vi "AMC Multiple Targets Example 1.vi"() -> ()   [LabVIEW 2017]
uses:
  Tools/Keyed Array/Tools_KeyedArray KeyedArray.ctl
panel:
  in  "Servers":i32(listbox)
  in  "Get All Queues":bool
  in  "Target IP Address":string="10.0.18.197"
  in  "Queue":string
  in  "Verify Queue":bool
  in  "PingAll":bool
  out "Response":string
  in  "Ping":bool
  in  "Exit":bool
  out "Process":bool
  in  "Process":bool
  out "Status":string
  in  "Process":bool
  in  "Exit":bool
  in  "State Variables":T1
  # "Target1"
  # "Local Messages >>"
  # "Remote Messages >>"
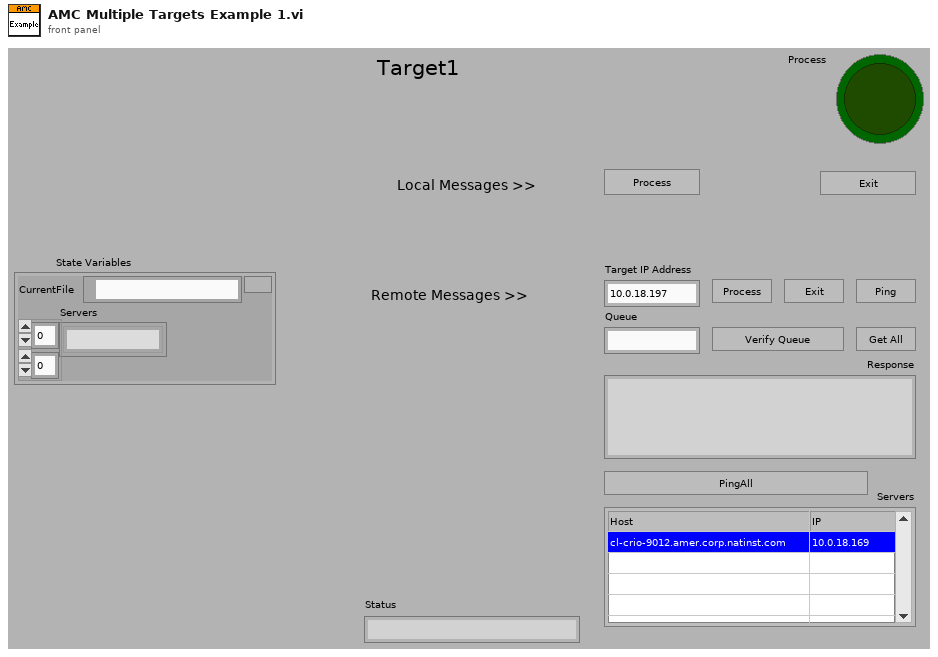
[diagram p1: front panel]
types:
  T1 = cluster{"CurrentFile":path, "Servers":string[][]}
  T2 = typedef "amc_Message Queue.ctl" = refnum<queue>
  T3 = typedef "Tools_KeyedArray KeyedArray.ctl" = cluster{"keys":string[], "values":string[]}
  T4 = typedef "LVPoint32TypeDef.ctl" = cluster{"Horizontal":i32, "Vertical":i32}
  T5 = typedef "LVRowAndColumnTypeDef.ctl" = cluster{"Row":i32, "Column":i32}
  T6 = typedef "amc_Message.ctl" = cluster{"Name":string, "Value":string, "Attributes":T3, "Receiver Host":string, "Receiver Process":string, "Source Host":string, "Source Process":string, "Priority Message":bool, "Acknowledge Message":bool}
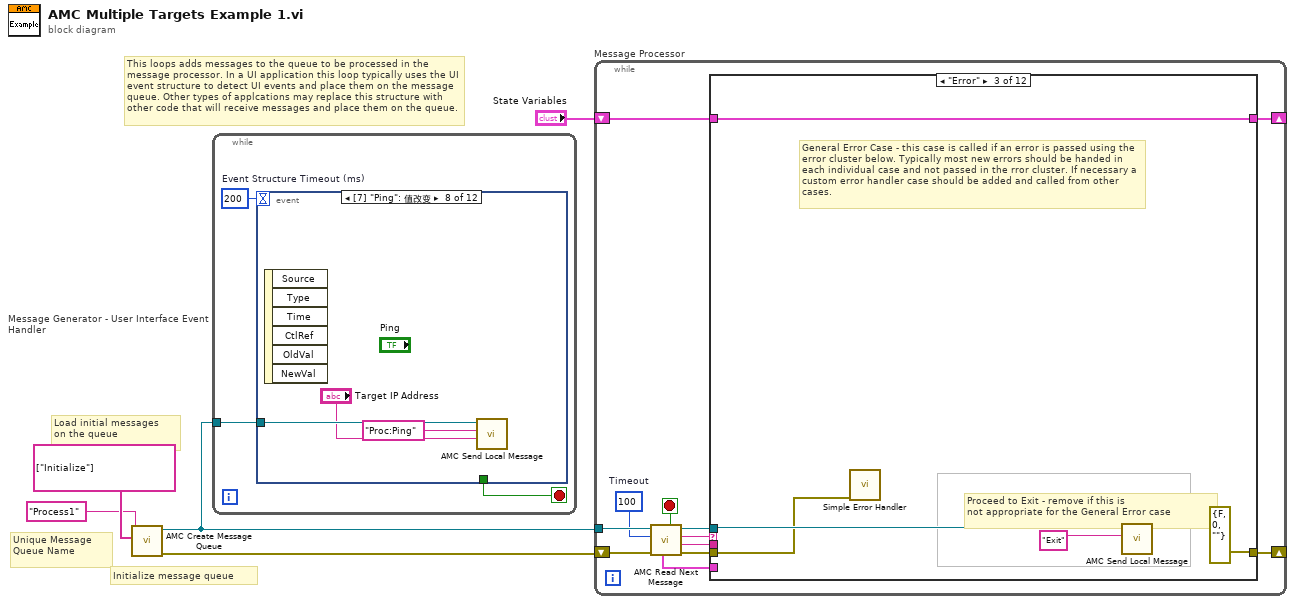
[diagram p0: block diagram]
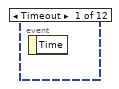
[diagram p2: hidden frame]
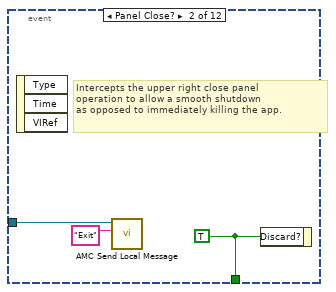
[diagram p3: hidden frame]
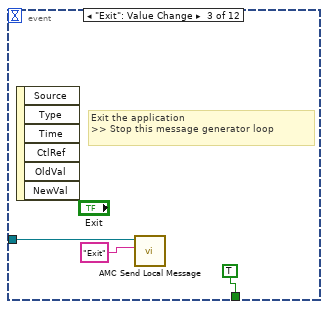
[diagram p4: hidden frame]
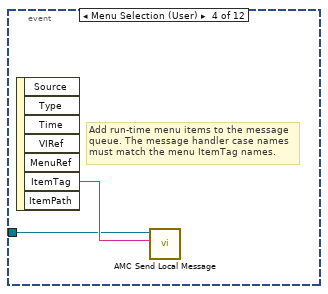
[diagram p5: hidden frame]
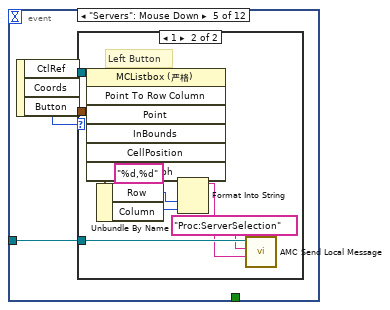
[diagram p6: hidden frame]
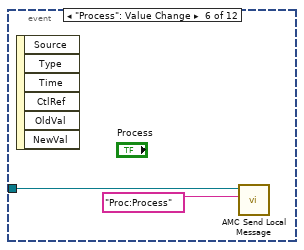
[diagram p8: hidden frame]
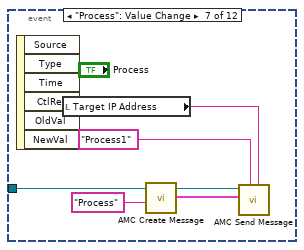
[diagram p9: hidden frame]
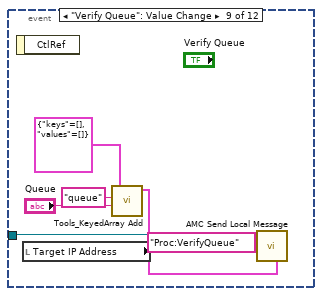
[diagram p10: hidden frame]
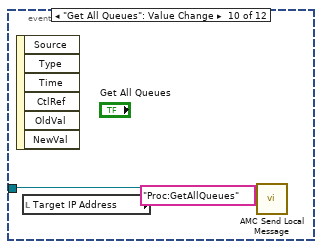
[diagram p11: hidden frame]
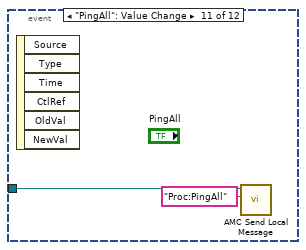
[diagram p12: hidden frame]
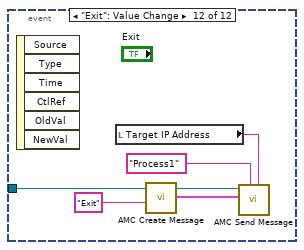
[diagram p13: hidden frame]
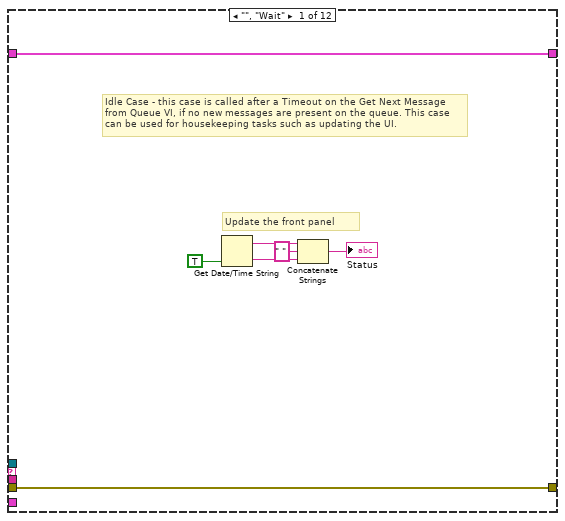
[diagram p14: hidden frame]
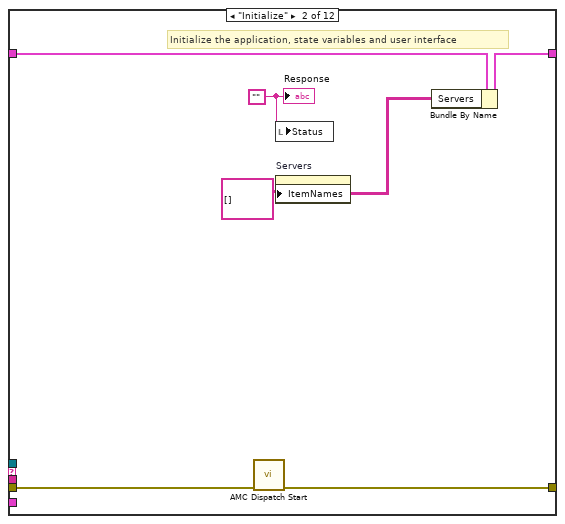
[diagram p15: hidden frame]
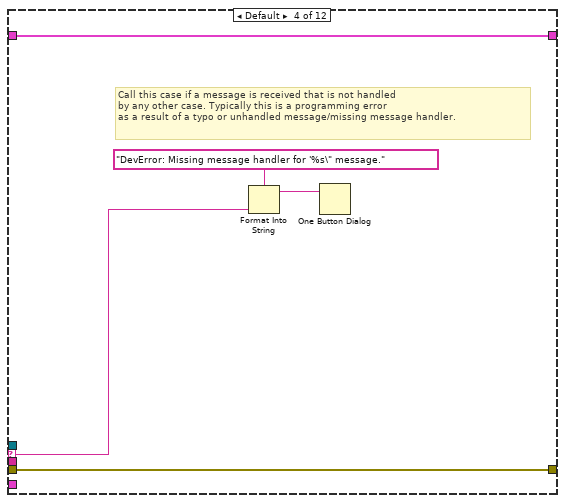
[diagram p16: hidden frame]
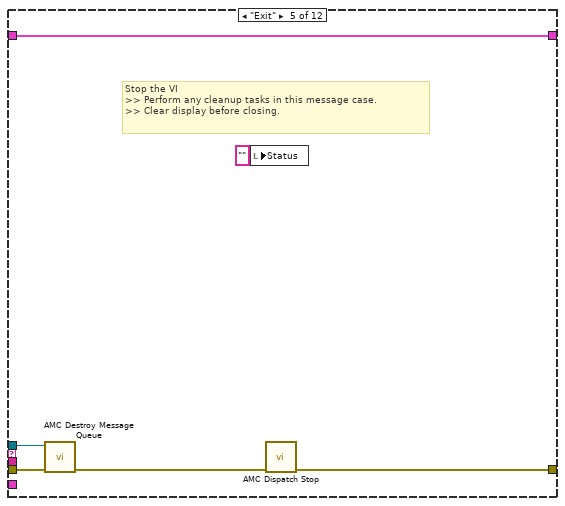
[diagram p17: hidden frame]
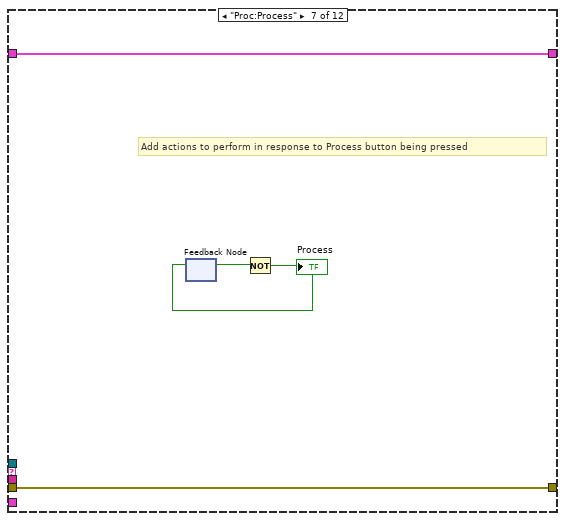
[diagram p19: hidden frame]
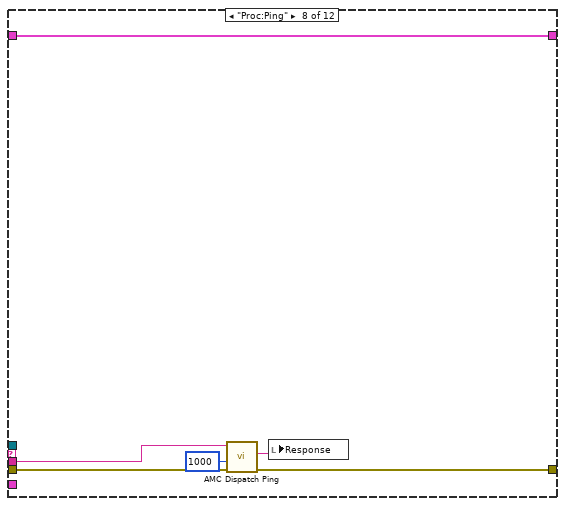
[diagram p20: hidden frame]
diagram:
  # "This loops adds messages to the queue to be processed in the message processor. In a UI application this loop typically uses the UI event structure to detect UI events and place them on the message queue. Other types of applcations may replace this structure with other code that will receive messages and place them on the queue."
  # "Initialize message queue"
  # "Unique Message\nQueue Name"
  # "Load initial messages\non the queue"
  n1 = call "AMC Create Message Queue.vi"("Initial Message Names"=string[] ["Initialize"], "Message Queue Name"="Process1" ("Message queue name (unnamed)")) -> ("error out"=w3:errorcluster, "Message Queue out"=w5:T2)  [unwired: 3 in, 5 out]
  n2 = while "Message Generator - User Interface Event Handler" {
    tunnel: w5 -> [w6]
    stop <- w7 stop-if-true
    w8 = 200  # Event Structure Timeout (ms)
    n3 = event shown="[7] \"Ping\": 值改变" {
      selector: _ -> [_ _ _ _ _ _ _ _ _ _ _ _]
      dyn-events: _ -> [_ _ _ _ _ _ _ _ _ _ _ _]
      timeout: w8 -> [_ _ _ _ _ _ _ _ _ _ _ _]
      tunnel: [_ w11 TRUE ("Discard?") _ _ _ _ _ _ _ _ _] -> w7
      tunnel: w6 -> [_ w9 w13 w15 w20 w31 w36 w39 w46 w49 w51 w56]
      event Timeout {
        n4 = event-data() -> ()  [unwired: 2 out]
      }
      event Panel Close? {
        w11 = TRUE ("Discard?")
        # "Intercepts the upper right close panel\noperation to allow a smooth shutdown\nas opposed to immediately killing the app."
        n5 = event-data() -> ()  [unwired: 4 out]
        n6 = call "AMC Send Local Message.vi"("Message Name"="Exit", "Message Queue in"=w9) -> ()  [unwired: 4 in, 6 out]
        n7 = event-data("Discard?"=w11) -> ()  [unwired: 1 in, 1 out]
      }
      event "Exit": Value Change {
        # "Exit the application\n>> Stop this message generator loop"
        n8 = event-data() -> ()  [unwired: 7 out]
        n9 = call "AMC Send Local Message.vi"("Message Name"="Exit", "Message Queue in"=w13) -> ()  [unwired: 4 in, 6 out]
      }
      event Menu Selection (User) {
        # "Add run-time menu items to the message\nqueue. The message handler case names must match the menu ItemTag names."
        n10 = event-data() -> ("ItemTag"=w16:string)  [unwired: 7 out]
        n11 = call "AMC Send Local Message.vi"("Message Name"=w16, "Message Queue in"=w15) -> ()  [unwired: 4 in, 6 out]
      }
      event "Servers": Mouse Down {
        n12 = event-data() -> ("CtlRef"=w19:refnum<vi>, "Coords"=w18:T4, "Button"=w17:u16)  [unwired: 1 out]
        n13 = case shown="1" w17 {
          tunnel: w20 -> [_ w29]
          tunnel: w19 -> [_ w27]
          tunnel: w18 -> [_ w26]
          frame Default {
          }
          frame 1 {
            # "Left Button"
            n14 = invoke class="MCListbox (严格)" method="Point To Row Column"(reference=w27, "Point"=w26) -> ("CellPosition"=w25:T5)  [unwired: 5 in, 6 out]
            n15 = Unbundle By Name(w25) -> ("Row"=w24:i32, "Column"=w23:i32)
            n16 = Format Into String(format string="%d,%d", w24, w23) -> (resulting string=w21:string)  [unwired: 2 in, 1 out]
            n17 = call "AMC Send Local Message.vi"("Message Value"=w21, "Message Name"="Proc:ServerSelection", "Message Queue in"=w29) -> ()  [unwired: 3 in, 6 out]
          }
        }
      }
      event "Process": Value Change {
        n18 = event-data() -> ()  [unwired: 7 out]
        n19 = call "AMC Send Local Message.vi"("Message Name"="Proc:Process", "Message Queue in"=w31) -> ()  [unwired: 4 in, 6 out]
      }
      event "Process": Value Change {
        n20 = event-data() -> ()  [unwired: 7 out]
        n21 = local read "Target IP Address"() -> (w32:string)
        n22 = call "AMC Create Message.vi"("Name"="Process") -> ("Message"=w34:T6)  [unwired: 2 in, 8 out]
        n23 = call "AMC Send Message.vi"("Receiver Host"=w32, "Receiver Process"="Process1" ("process"), "Message"=w34, "Message Queue in"=w36) -> ()  [unwired: 4 in, 4 out]
      }
      event "Ping": Value Change {
        n24 = event-data() -> ()  [unwired: 7 out]
        n25 = call "AMC Send Local Message.vi"("Message Value"="Target IP Address", "Message Name"="Proc:Ping", "Message Queue in"=w39) -> ()  [unwired: 3 in, 6 out]
      }
      event "Verify Queue": Value Change {
        n26 = event-data() -> ()  [unwired: 2 out]
        n27 = local read "Target IP Address"() -> (w44:string)
        n28 = call "Tools_KeyedArray Add.vi"("value"="Queue", "key"="queue", "array in"=T3 {"keys"=[], "values"=[]}) -> ("array out"=w40:T3)  [unwired: 1 in, 3 out]
        n29 = call "AMC Send Local Message.vi"("Message Attributes"=w40, "Message Value"=w44, "Message Name"="Proc:VerifyQueue", "Message Queue in"=w46) -> ()  [unwired: 3 in, 5 out]
      }
      event "Get All Queues": Value Change {
        n30 = event-data() -> ()  [unwired: 7 out]
        n31 = local read "Target IP Address"() -> (w47:string)
        n32 = call "AMC Send Local Message.vi"("Message Value"=w47, "Message Name"="Proc:GetAllQueues", "Message Queue in"=w49) -> ()  [unwired: 3 in, 6 out]
      }
      event "PingAll": Value Change {
        n33 = event-data() -> ()  [unwired: 7 out]
        n34 = call "AMC Send Local Message.vi"("Message Name"="Proc:PingAll", "Message Queue in"=w51) -> ()  [unwired: 4 in, 6 out]
      }
      event "Exit": Value Change {
        n35 = event-data() -> ()  [unwired: 7 out]
        n36 = local read "Target IP Address"() -> (w53:string)
        n37 = call "AMC Create Message.vi"("Name"="Exit") -> ("Message"=w54:T6)  [unwired: 2 in, 8 out]
        n38 = call "AMC Send Message.vi"("Receiver Host"=w53, "Receiver Process"="Process1" ("process"), "Message"=w54, "Message Queue in"=w56) -> ()  [unwired: 4 in, 4 out]
      }
    }
  }
  n39 = while "Message Processor" {
    shift-left: w3 -> [w63]
    shift-right: [w64] -> _
    tunnel: w5 -> [w62]
    shift-left: "State Variables" -> [w68]
    shift-right: [w67] -> _
    stop <- w61 stop-if-true
    w60 = 100  # Timeout
    n40 = call "AMC Read Next Message.vi"("error in (no error)"=w63, "timeout (1ms)"=w60, "Message Queue in"=w62) -> ("error out"=w65:errorcluster, "Message Value"=w57:string, "Message Name"=w59:string, "Message Queue out"=w66:T2, "Exit Process"=w61:bool, "Message"=w58:T6)  [unwired: 1 in, 2 out]
    n41 = case shown="\"Error\"" w59 {
      selector: w59 -> [_ _ _ w89 _ _ _ _ _ _ _ _]
      tunnel: [w75 w77 w86 w91 w96 w99 w102 w109 w111 w133 w138 w146] -> w67
      tunnel: w68 -> [w75 w78 w86 w91 w96 w99 w102 w109 w112 w133 w138 w146]
      tunnel: w66 -> [_ _ w84 _ w94 _ _ _ _ _ _ _]
      tunnel: w65 -> [w74 w80 w83 w90 w97 w98 w103 w108 w117 w126 w135 w145]
      tunnel: [w74 w79 errorcluster {"status"=FALSE, "code"=0, "source"=""} ("error out") w90 w92 w98 w103 w107 w116 w125 w134 w145] -> w64
      tunnel: w58 -> [_ _ _ _ _ _ _ _ _ w132 _ _]
      tunnel: w57 -> [_ _ _ _ _ _ _ w105 _ w129 w137 w142]
      frame "", "Wait" {
        # "Update the front panel"
        # "Idle Case - this case is called after a Timeout on the Get Next Message from Queue VI, if no new messages are present on the queue. This case can be used for housekeeping tasks such as updating the UI."
        n42 = Get Date/Time String(want seconds? (F)=TRUE) -> (date string=w73:string, time string=w72:string)  [unwired: 2 out]
        n43 = Concatenate Strings(w73, " " ("string"), w72) -> (→"Status":string)
      }
      frame "Initialize" {
        w76 = string[][] [] ("Item Names")
        w81 = ""
        # "Initialize the application, state variables and user interface"
        n44 = call "AMC Dispatch Start.vi"("error in (no error)"=w80) -> ("error out"=w79:errorcluster)  [unwired: 1 in, 9 out]
        n45 = local write "Status"(w81) -> ()
        n46 = property on="Servers" class="MCListbox (严格)"("ItemNames"=w76) -> ()  [unwired: 2 in, 2 out]
        n47 = Bundle By Name(cluster=w78, "Servers"=w76) -> (w77:T1)
        "Response" <- w81
      }
      frame "Error" {
        # "Proceed to Exit - remove if this is\nnot appropriate for the General Error case"
        # "General Error Case - this case is called if an error is passed using the error cluster below. Typically most new errors should be handed in each individual case and not passed in the rror cluster. If necessary a custom error handler case should be added and called from other cases."
        n48 = call <vilib>:"Simple Error Handler.vi"("error in (no error)"=w83) -> ()  [unwired: 1 in, 8 out]
        n49 = call "AMC Send Local Message.vi"("Message Name"="Exit", "Message Queue in"=w84) -> ()  [unwired: 4 in, 6 out]
      }
      frame Default {
        # "Call this case if a message is received that is not handled \nby any other case. Typically this is a programming error\nas a result of a typo or unhandled message/missing message handler."
        n50 = Format Into String(format string="DevError: Missing message handler for '%s\" message." ("message"), w89) -> (resulting string=w87:string)  [unwired: 2 in, 1 out]
        n51 = One Button Dialog(message=w87) -> ()  [unwired: 2 out]
      }
      frame "Exit" {
        # "Stop the VI\n>> Perform any cleanup tasks in this message case.\n>> Clear display before closing."
        n52 = call "AMC Destroy Message Queue.vi"("error in (no error)"=w97, "Message Queue in"=w94) -> ("error out"=w93:errorcluster)  [unwired: 9 out]
        n53 = local write "Status"("" ("Status")) -> ()
        n54 = call "AMC Dispatch Stop.vi"("error in (no error)"=w93) -> ("error out"=w92:errorcluster)  [unwired: 10 out]
      }
      frame "**** App Processing Functions ****" {
      }
      frame "Proc:Process" {
        # "Add actions to perform in response to Process button being pressed"
        n55 = feedback #1() -> (w101:bool)  [unwired: 1 out]
        n56 = Not(x=w101) -> (.not. x?=w100:bool)
        "Process" <- w100
        n57 = feedback-in #1(w100) -> ()
      }
      frame "Proc:Ping" {
        n58 = call "AMC Dispatch Ping.vi"("error in (no error)"=w108, "Timeout (100 ms)"=1000, "receiver host"=w105) -> ("error out"=w107:errorcluster, "String Response"=w106:string)  [unwired: 7 out]
        n59 = local write "Response"(w106) -> ()
      }
      frame "Proc:PingAll" {
        n60 = call "AMC Dispatch PingAll.vi"("error in (no error)"=w117, "Timeout (1000 ms)"=1000) -> ("error out"=w116:errorcluster, "Response"=w115:string, "Messages"=w113:T6[])  [unwired: 2 in, 5 out]
        n61 = for {
          tunnel: w113 -> [w123] mode=indexing
          tunnel: [w118] -> w110 mode=indexing
          n62 = Unbundle By Name(w123) -> ("Source Host"=w120:string, "Attributes"=w122:T3)
          n63 = call "Tools_KeyedArray Index.vi"("key"="IP", "array in"=w122) -> ("value"=w119:string)  [unwired: 2 in, 3 out]
          n64 = Build Array(w120, w119) -> (w118:string[])
        }
        n65 = local write "Response"(w115) -> ()
        n66 = property on="Servers" class="MCListbox (严格)"("ItemNames"=w110) -> ()  [unwired: 2 in, 2 out]
        n67 = Bundle By Name(cluster=w112, "Servers"=w110) -> (w111:T1)
      }
      frame "Proc:VerifyQueue" {
        n68 = Unbundle By Name(w132) -> ("Attributes"=w131:T3)
        n69 = call "Tools_KeyedArray Index.vi"("key"="queue", "array in"=w131) -> ("value"=w128:string)  [unwired: 2 in, 3 out]
        n70 = call "AMC Dispatch Verify Queue.vi"("error in (no error)"=w126, "Timeout (100 ms)"=1000, "queue name"=w128, "receiver host"=w129) -> ("error out"=w125:errorcluster, "String Response"=w127:string)  [unwired: 6 out]
        n71 = local write "Response"(w127) -> ()
      }
      frame "Proc:GetAllQueues" {
        n72 = call "AMC Dispatch Get All Queues.vi"("error in (no error)"=w135, "receiver host"=w137) -> ("error out"=w134:errorcluster, "String Response"=w136:string)  [unwired: 1 in, 7 out]
        n73 = local write "Response"(w136) -> ()
      }
      frame "Proc:ServerSelection" {
        n74 = Unbundle By Name(w146) -> ("Servers"=w144:string[][])
        n75 = Scan From String(format string="%d,%d", input string=w142) -> (output 1=w140:i32, output 2=w139:i32)  [unwired: 2 in, 5 out]
        n76 = Index Array(array=w144, index (row)=w140, index (col)=w139) -> (element=w143:string)
        n77 = local write "Target IP Address"(w143) -> ()
      }
    }
  }
